vi "Record and playback example for pco.cameras with CamRam.vi"() -> ()   [LabVIEW 2012]
doc: "A short program to demonstrate the fundamentals of control and image acquision for pco.camera models with internal camRAM memory, such as the pco.dimax or pco.1200. The program records a sequence of images, with \"live\" updating, until the \"StopRecording\" button is pressed. A subset of recorded images is then read out from the camera RAM. WARNING: Limit the number of images read back tfrom the camera RAM to a reasonable number. Images are stored as a three-dimensional array, which can very large. Use ctrl-H for more help on the individual controls and indicators."
panel:
  in  "Rate":i32(ring) items=["12000000", "24000000"]
  out "bClose":bool
  in  "Quit":bool
  in  "ImageNr":i32
  in  "Image":i32
  out "BufNr1":i16
  out "BufNr0":i16
  in  "bUseBuffer1":bool
  in  "bUseBuffer0":bool
  in  "ROIX1":u16=1 min=1
  in  "ROIY1":u16=1 min=1
  in  "ROIY0":u16=1 min=1
  in  "ROIX0":u16=1 min=1
  out "Bits/pixel":u16
  in  "Readout":bool
  in  "Record":bool
  in  "Stop":u32=10 min=1
  in  "Start":u32=1 min=1
  in  "DelayTimeBase":u16(ring)=2 items=["nanoseconds", "microseconds", "milliseconds"]
  in  "ExposureTimeBase":u16(ring)=2 items=["nanoseconds", "microseconds", "milliseconds"]
  in  "Exposure":u32=10
  in  "Delay":u32
  out "Reading":bool
  in  "StorageMode":bool
  out "ImageCount":u32
  out "Image":u16[][](graph)
  in  "TriggerMode":u16(ring) items=["Auto", "Software", "External sequence start ", "External exposure control"]
  # "A short program to demonstrate the fundamentals of control and image acquision for pco.camera models with internal camRAM memory, such as the pco.dimax or pco.1200. The program records a sequence of images, with \"live\" updating, until the \"StopRecording\" button is pressed. A subset of recorded images is then read out from the camera RAM. WARNING: Limit the number of images read back tfrom the camera RAM to a reasonable number. Images are stored as a three-dimensional array, which can very large.  Use ctrl-H for more help on the individual controls and indicators."
  # "pco.labview"
  # "1) Setup camera:"
  # "FIFO"
  # "Recorder"
  # "2) Record  images:"
  # "3) Read out images:"
  # "4) Display image:"
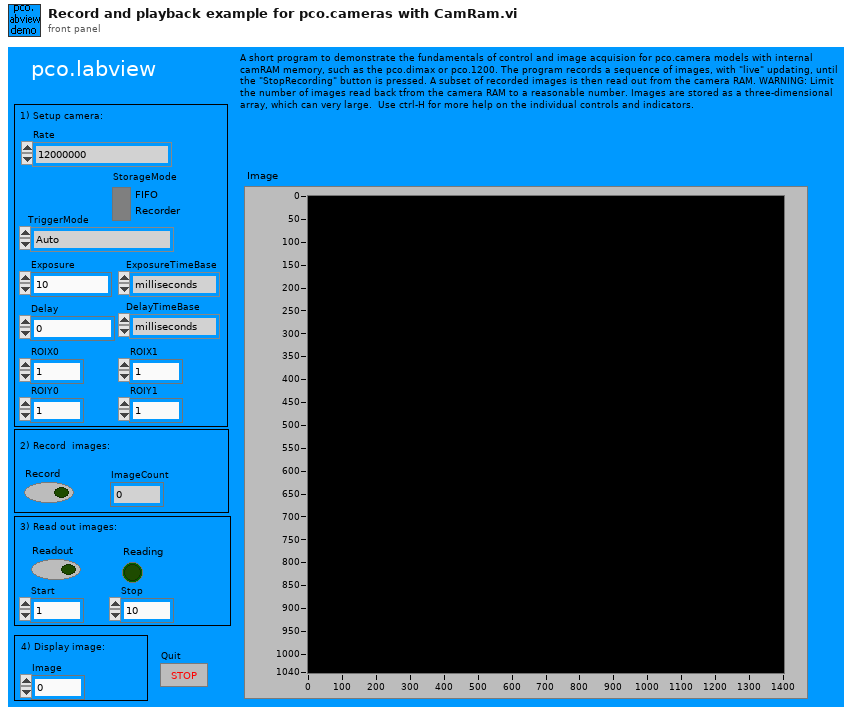
[diagram p1: front panel]
types:
  T1 = cluster{"SSize":u16, "CamType":u16, "CamsSubType":u16, "SerialNumber":u32, "HWVersion":u32, "FWVersion ":u32, "InterfaceType":u16, "HardwareVersions":cluster{"Board":u16, cluster{"string":string, "BatchNumber":u16, "MinorRevision":u8, "MajorRevision":u8, "Variant":u16}[]}, "FirmwareVersions":cluster{"DeviceNum":u16, cluster{"string":string, "MinorRevision":u8, "MajorRevision":u8, "Variant":u16}[]}}
  T2 = cluster{"Size":u16, "SensorTypeDESC":u16, "SensorSubtypeDESC":u16, "MaxHorizontalResStdDESC":u16, "MaxVerticalResStdDESC":u16, "MaxHorizontalResExtDESC":u16, "MaxVerticalResExtDESC":u16, "DynResDESC":u16, "MaxBinHorzDESC":u16, "BinHorzStepDESC":bool, "MaxBinVertDESC":u16, "BinVertStepDESC":bool, "ROIHorzStepDESC":u16, "ROIVertStepDESC":u16, "NumADCDESC":u16, "IRDESC":bool, "MinDelayDESC":u32, "MaxDelayDESC":u32, "MinDelayStepDESC":u32, "MinExpoDESC":u32, "MaxExpoDESC":u32, "MinExpoStepDESC":u32, "MinDelayIRDESC":u32, "MaxDelayIRDESC":u32, "MinExpoIRDESC":u32, "MaxExpoIRDESC":u32, "TimeTableDESC":bool, "DoubleImageDESC":bool, "MinCoolSetDESC":i16, "MaxCoolSetDESC":i16, "MDefaultCoolSetDESC":i16, "PowerDownModeDESC":bool, "OffsetRegDESC":bool, "ColorPattern":cluster{"UpperLeftColor":u8, "UpperRightColor":u8, "LowerLeftColor":u8, "LowerRightColor":u8}, "PatternTypeDESC":bool, "PixelRates":u32[], "CoversionFactors":u16[], "Reserved":u32[], "GeneralCapabilities":u32, "GeneralCapabilities 2":u32, "Min Size Hor":u16, "Min Size Vert":u16, "Ext Synch Freq":u32[], "Cooling Setpoints":i16[], "Soft ROI Hor Step":u16, "Soft ROI Vert Step":u16}
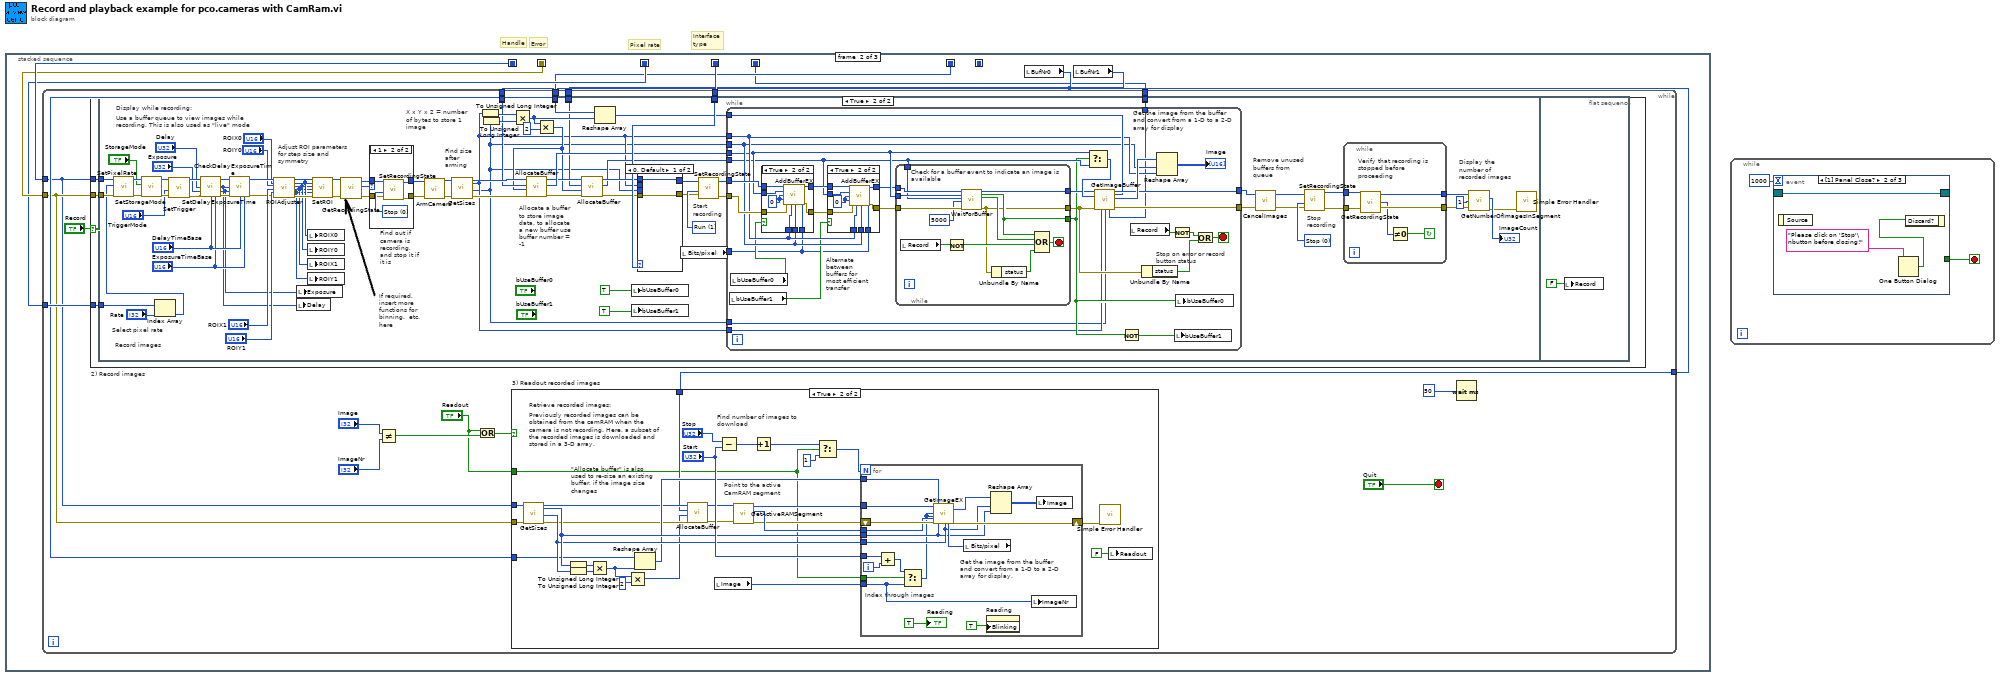
[diagram p0: block diagram]
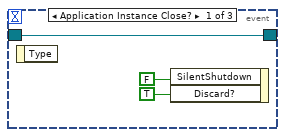
[diagram p2: hidden frame]
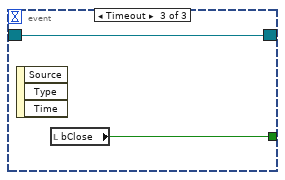
[diagram p3: hidden frame]
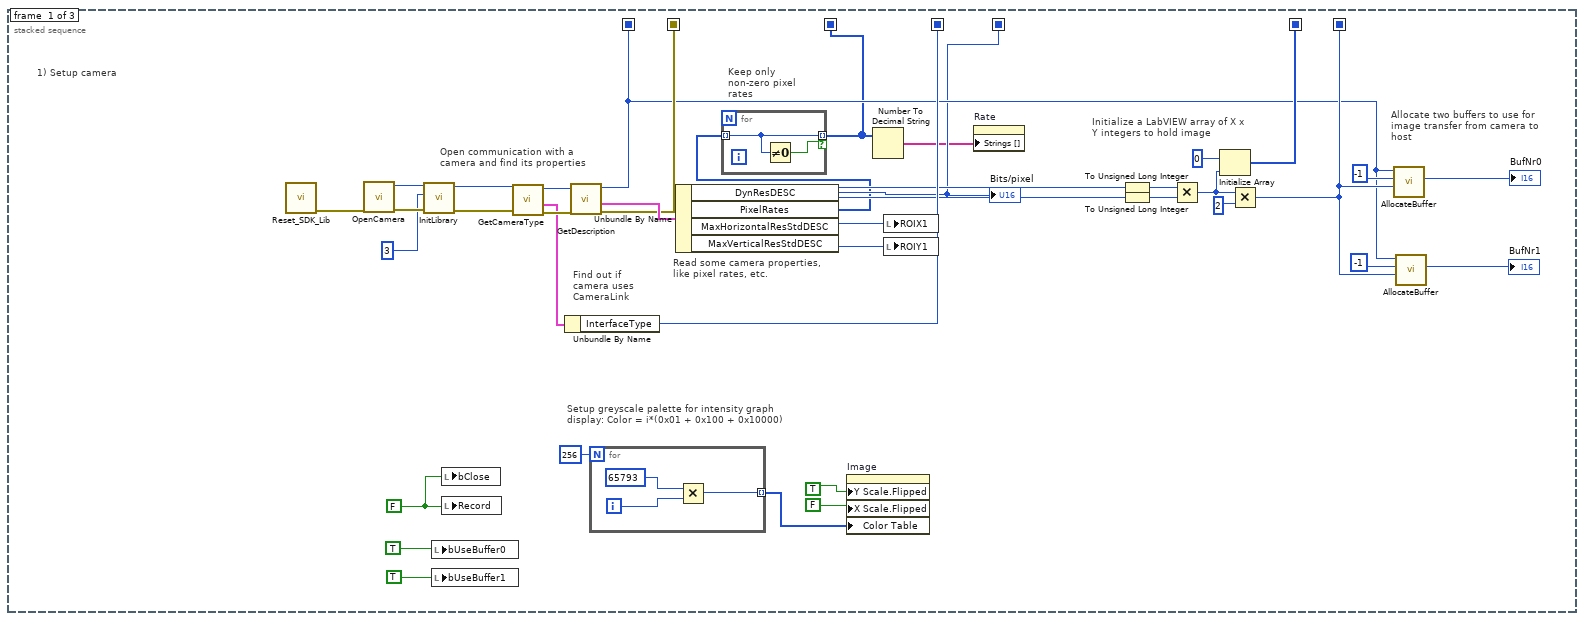
[diagram p4: hidden frame]
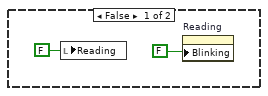
[diagram p5: hidden frame]
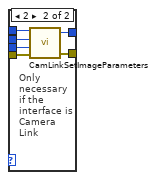
[diagram p9: hidden frame]
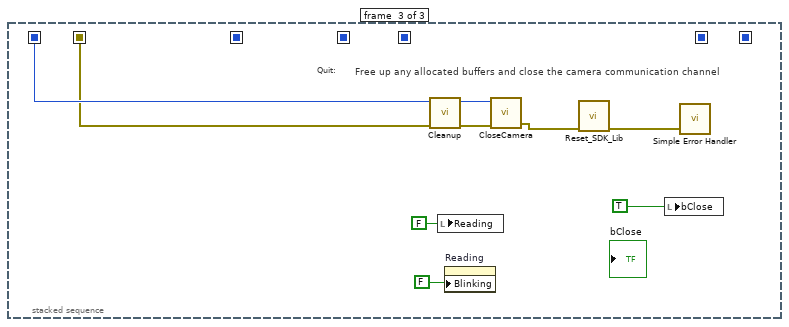
[diagram p11: hidden frame]
diagram:
  # "Interface type"
  # "Error"
  # "Handle"
  # "Pixel rate"
  n1 = stacked-sequence {
    seq-local: [w31 _ _] -> [_ w46 _]
    seq-local: [w18 _ _] -> [_ _ _]
    seq-local: [w1 _ _] -> [_ w48 _]
    seq-local: [w17 _ _] -> [_ w50 w299]
    seq-local: [w25 _ _] -> [_ w49 w298]
    seq-local: [w24 _ _] -> [_ w47 _]
    seq-local: [w4 _ _] -> [_ w43 _]
    frame #0 {
      w11 = FALSE ("stop")
      # "Keep only non-zero pixel rates"
      # "Read some camera properties, like pixel rates, etc."
      # "Allocate two buffers to use for image transfer from camera to host"
      # "1) Setup camera"
      # "Find out if camera uses CameraLink"
      # "Setup greyscale palette for intensity graph display: Color = i*(0x01 + 0x100 + 0x10000)"
      # "Initialize a LabVIEW array of X x Y integers to hold image"
      # "Open communication with a camera and find its properties"
      n2 = call "Reset_SDK_Lib.vi"() -> ("ErrorOut"=w7:errorcluster)  [unwired: 11 in]
      n3 = call "OpenCamera.vi"("ErrorIn"=w7) -> ("ErrorOut"=w9:errorcluster, "Handle out"=w10:u64)  [unwired: 3 in, 2 out]
      n4 = call "InitLibrary.vi"("error in (no error)"=w9, "InterfaceType"=u32 3, "ph"=w10) -> ("error out"=w5:errorcluster, "hout"=w6:u64)  [unwired: 7 in]
      n5 = local write "bUseBuffer0"(TRUE) -> ()
      n6 = local write "bUseBuffer1"(TRUE) -> ()
      n7 = local write "bClose"(w11) -> ()
      n8 = local write "Record"(w11) -> ()
      n9 = call "GetCameraType.vi"("ph"=w6, "error in (no error)"=w5) -> ("hout"=w28:u64, "CameraType"=w26:T1, "error out"=w27:errorcluster)  [unwired: 1 in, 1 out]
      n10 = Unbundle By Name(w26) -> ("InterfaceType"=w24:u16)
      n11 = call "GetDescription.vi"("ErrorIn"=w27, "ph"=w28) -> ("ErrorOut"=w25:errorcluster, "Description"=w30:T2, "hout"=w17:u64)  [unwired: 2 in, 1 out]
      n12 = for {
        N: 256 -> [_]
        tunnel: [w40] -> w34 mode=indexing
        i -> [w41]
        n13 = Multiply(x=65793, y=w41) -> (x*y=w40:i32)
      }
      n14 = Unbundle By Name(w30) -> ("DynResDESC"=w4:u16, "PixelRates"=w2:u32[], "MaxHorizontalResStdDESC"=w23:u16, "MaxVerticalResStdDESC"=w22:u16)
      "Bits/pixel" <- w4
      n15 = for {
        tunnel: w2 -> [w39] mode=indexing
        tunnel: [w39] -> w1 mode=indexing if=w38
        n16 = Not Equal To 0?(x=w39) -> (x != 0?=w38:bool)
      }
      n17 = property on="Image" class="IntGraph (strict)"("Y Scale.Flipped"=TRUE, "X Scale.Flipped"=FALSE, "Color Table"=w34) -> ()  [unwired: 2 in, 2 out]
      n18 = Number To Decimal String(number=w1) -> (decimal integer string=w3:string[])  [unwired: 1 in]
      n19 = local write "ROIX1"(w23) -> ()
      n20 = local write "ROIY1"(w22) -> ()
      n21 = property on="Rate" class="Ring (strict)"("Strings []"=w3) -> ()  [unwired: 2 in, 2 out]
      n22 = To Unsigned Long Integer(number=w23) -> (unsigned 32bit integer=w20:u32)
      n23 = To Unsigned Long Integer(number=w22) -> (unsigned 32bit integer=w19:u32)
      n24 = Multiply(x=w20, y=w19) -> (x*y=w32:u32)
      n25 = Initialize Array(u16 0 ("Element Data"), w32) -> (w31:u16[])
      n26 = Multiply(x=w32, y=u32 2) -> (x*y=w18:u32)
      n27 = call "AllocateBuffer.vi"("Size"=w18, "BufNr"=i16 -1, "ph"=w17) -> ("BufNrOut"=→"BufNr0":i16)  [unwired: 3 in, 5 out]
      n28 = call "AllocateBuffer.vi"("Size"=w18, "BufNr"=-1, "ph"=w17) -> ("BufNrOut"=→"BufNr1":i16)  [unwired: 3 in, 5 out]
    }
    frame #1 {
      n29 = local read "BufNr0"() -> (w45:i16)
      n30 = local read "BufNr1"() -> (w44:i16)
      n31 = while {
        tunnel: w45 -> [w60]
        tunnel: w45 -> [w61]
        tunnel: w46 -> [w63]
        tunnel: w47 -> [w64]
        tunnel: w48 -> [w65]
        tunnel: w49 -> [w62]
        tunnel: w50 -> [w58]
        tunnel: w44 -> [w59]
        tunnel: w43 -> [w51]
        stop <- "Quit" stop-if-true
        n32 = case "2) Record images" shown="True" "Record" {
          tunnel: w58 -> [_ w124]
          tunnel: w62 -> [_ w123]
          tunnel: w65 -> [_ w122]
          tunnel: w64 -> [_ w121]
          tunnel: w63 -> [_ w120]
          tunnel: w61 -> [_ w119]
          tunnel: w59 -> [_ w118]
          tunnel: w51 -> [_ w117]
          frame False {
          }
          frame True {
            n33 = flat-sequence {
              tunnel: w124 -> [w186]
              tunnel: w123 -> [w185]
              tunnel: w122 -> [w147]
              tunnel: w121 -> [w183]
              tunnel: w120 -> [w181]
              tunnel: w119 -> [w171]
              tunnel: w118 -> [w165]
              tunnel: w117 -> [w149]
              frame #0 {
                w204 = u16 1 items=["Stop", "Run"] ("RecordingState")
                w207 = u16 0 items=["Stop", "Run"] ("RecordingState")
                # "Adjust ROI parameters   for step size and symmetry"
                # "Select pixel rate"
                # "Remove unused buffers from queue"
                # "Display the number of recorded images"
                # "Record images"
                # "Start recording"
                # "Allocate a buffer to store image data. to allocate a new buffer use buffer number = -1"
                # "Find size after arming"
                # "Find out if camera is recording, and stop it if it is"
                # "If required, insert more functions for binning.  etc. here"
                # "X x Y x 2 = number of bytes to store 1 image"
                # "Stop recording"
                # "Use a buffer queue to view images while recording. This is also used as \"live\" mode"
                # "Display while recording:"
                n34 = Index Array(array=w147, index="Rate") -> (element=w146:u32)
                n35 = call "SetPixelRate.vi"("error in (no error)"=w185, "PixelRate"=w146, "ph"=w186) -> ("error out"=w202:errorcluster, "hout"=w203:u64)  [unwired: 2 in, 1 out]
                n36 = call "SetStorageMode.vi"("error in (no error)"=w202, "StorageMode"="StorageMode", "ph"=w203) -> ("error out"=w194:errorcluster, "hout"=w195:u64)  [unwired: 2 in, 1 out]
                n37 = call "SetTrigger.vi"("error in (no error)"=w194, "TriggerMode"="TriggerMode", "ph"=w195) -> ("error out"=w134:errorcluster, "hout"=w131:u64)  [unwired: 2 in, 1 out]
                n38 = call "CheckDelayExposureTime.vi"("ph"=w131, "Delay"="Delay", "Exposure"="Exposure", "error in (no error)"=w134, "DelayTimeBase"="DelayTimeBase", "ExposureTimeBase"="ExposureTimeBase") -> ("hout"=w132:u64, "Delay Out"=w126:u32, "Exposure Out"=w125:u32, "error out"=w133:errorcluster)  [unwired: 4 in, 2 out]
                n39 = call "SetDelayExposureTime.vi"("ph"=w132, "Delay"=w126, "Exposure"=w125, "error in (no error)"=w133, "DelayTimeBase"="DelayTimeBase", "ExposureTimeBase"="ExposureTimeBase") -> ("hout"=w174:u64, "error out"=w140:errorcluster)  [unwired: 7 in, 1 out]
                n40 = call "ROIAdjuster.vi"("HandleIn"=w174, "ROIXmin"="ROIX0", "ROIYmin"="ROIY0", "ROIXmax"="ROIX1", "ROIYmax"="ROIY1", "ErrorIn"=w140) -> ("hout"=w145:u64, "ROIX0Mod"=w138:u16, "ROIY0Mod"=w137:u16, "ROIX1Mod"=w136:u16, "ROIY1Mod"=w135:u16, "ErrorOut"=w139:errorcluster)  [unwired: 7 in, 1 out]
                n41 = local write "Delay"(w126) -> ()
                n42 = local write "Exposure"(w125) -> ()
                n43 = local write "ROIX0"(w138) -> ()
                n44 = local write "ROIY0"(w137) -> ()
                n45 = local write "ROIX1"(w136) -> ()
                n46 = local write "ROIY1"(w135) -> ()
                n47 = call "SetROI.vi"("ph"=w145, "ROIX0"=w138, "ROIY0"=w137, "ROIX1"=w136, "ROIY1"=w135, "error in (no error)"=w139) -> ("hout"=w173:u64, "error out"=w172:errorcluster)  [unwired: 12 in]
                n48 = call "GetRecordingState.vi"("ErrorIn"=w172, "ph"=w173) -> ("ErrorOut"=w198:errorcluster, "RecordingState"=w200:u16, "hout"=w199:u64)  [unwired: 2 in, 1 out]
                n49 = case shown="1" w200 {
                  tunnel: w199 -> [w288 w292]
                  tunnel: w198 -> [w287 w291]
                  tunnel: [w288 w290] -> w197
                  tunnel: [w287 w289] -> w196
                  frame 0, Default {
                  }
                  frame 1 {
                    w293 = u16 0 items=["Stop", "Run"] ("RecordingState")
                    n50 = call "SetRecordingState.vi"("ErrorIn"=w291, "RecordingState"=w293, "ph"=w292) -> ("ErrorOut"=w289:errorcluster, "hout"=w290:u64)  [unwired: 2 in, 1 out]
                  }
                }
                n51 = call "ArmCamera.vi"("error in (no error)"=w196, "ph"=w197) -> ("error out"=w192:errorcluster, "hout"=w193:u64)  [unwired: 1 in, 1 out]
                n52 = call "GetSizes.vi"("ph"=w193, "ErrorIn"=w192) -> ("hout"=w189:u64, "XResAct"=w151:u16, "YResAct"=w150:u16, "ErrorOut"=w191:errorcluster)  [unwired: 11 in, 3 out]
                n53 = To Unsigned Long Integer(number=w151) -> (unsigned 32bit integer=w175:u32)
                n54 = To Unsigned Long Integer(number=w150) -> (unsigned 32bit integer=w176:u32)
                n55 = Multiply(x=w175, y=w176) -> (x*y=w177:u32)
                n56 = Multiply(x=w177, y=u32 2) -> (x*y=w166:u32)
                n57 = call "AllocateBuffer.vi"("error in (no error)"=w191, "Size"=w166, "BufNr"=w171, "ph"=w189) -> ("error out"=w170:errorcluster, "BufNrOut"=w178:i16, "hout"=w168:u64)  [unwired: 2 in, 3 out]
                n58 = call "AllocateBuffer.vi"("error in (no error)"=w170, "Size"=w166, "BufNr"=w165, "ph"=w168) -> ("error out"=w169:errorcluster, "BufNrOut"=w164:i16, "hout"=w167:u64)  [unwired: 2 in, 3 out]
                n59 = Reshape Array(w181, w177) -> (w180:u16[])
                n60 = local write "bUseBuffer0"(TRUE) -> ()
                n61 = local write "bUseBuffer1"(TRUE) -> ()
                n62 = case shown="0, Default" w183 {
                  tunnel: w169 -> [w279 w286]
                  tunnel: [w279 w285] -> w188
                  tunnel: w167 -> [w280 w284]
                  tunnel: [w280 w283] -> w187
                  tunnel: w150 -> [_ w282]
                  tunnel: w151 -> [_ w281]
                  frame 0, Default {
                  }
                  frame 2 {
                    # "Only necessary if the interface is Camera Link"
                    n63 = call "CamLinkSetImageParameters.vi"("error in (no error)"=w286, "YRes"=w282, "XRes"=w281, "ph"=w284) -> ("error out"=w285:errorcluster, "hout"=w283:u64)  [unwired: 1 out]
                  }
                }
                n64 = local read "Bits/pixel"() -> (w157:u16)
                n65 = call "SetRecordingState.vi"("ErrorIn"=w188, "RecordingState"=w204, "ph"=w187) -> ("ErrorOut"=w184:errorcluster, "hout"=w182:u64)  [unwired: 2 in, 1 out]
                n66 = while {
                  tunnel: w178 -> [w220]
                  tunnel: w180 -> [w233]
                  tunnel: w182 -> [w232]
                  tunnel: w150 -> [w227]
                  tunnel: w151 -> [w228]
                  tunnel: w184 -> [w230]
                  tunnel: [w235] -> w156
                  tunnel: [w236] -> w155
                  tunnel: w164 -> [w219]
                  tunnel: w157 -> [w223]
                  tunnel: w151 -> [w210]
                  tunnel: w150 -> [w209]
                  tunnel: w149 -> [w208]
                  stop <- w211 stop-if-true
                  # "Alternate between buffers for most efficient transfer"
                  # "Stop on error or record button status"
                  # "Get the image from the buffer and convert from a 1-D to a 2-D array for display"
                  n67 = local read "bUseBuffer1"() -> (w225:bool)
                  n68 = local read "bUseBuffer0"() -> (w226:bool)
                  n69 = case shown="True" w226 {
                    tunnel: [w239 w248] -> w229
                    tunnel: [w238 w247] -> w231
                    tunnel: w220 -> [_ w246]
                    tunnel: w232 -> [w238 w245]
                    tunnel: w223 -> [_ w243]
                    tunnel: w228 -> [_ w242]
                    tunnel: w227 -> [_ w241]
                    tunnel: w230 -> [w239 w240]
                    frame False {
                    }
                    frame True {
                      w244 = 0
                      n70 = call "AddBufferEX.vi"("ph"=w245, "BuffNr"=w246, "1stImage"=w244, "LastImage"=w244, "error in (no error)"=w240, "XRes"=w242, "YRes"=w241, "BitPerPixel"=w243) -> ("hout"=w247:u64, "error out"=w248:errorcluster)  [unwired: 5 in, 1 out]
                    }
                  }
                  n71 = case shown="True" w225 {
                    tunnel: [w249 w259] -> w217
                    tunnel: [w250 w258] -> w218
                    tunnel: w219 -> [_ w257]
                    tunnel: w231 -> [w250 w256]
                    tunnel: w223 -> [_ w254]
                    tunnel: w228 -> [_ w253]
                    tunnel: w227 -> [_ w252]
                    tunnel: w229 -> [w249 w251]
                    frame False {
                    }
                    frame True {
                      w255 = 0
                      n72 = call "AddBufferEX.vi"("ph"=w256, "BuffNr"=w257, "1stImage"=w255, "LastImage"=w255, "error in (no error)"=w251, "XRes"=w253, "YRes"=w252, "BitPerPixel"=w254) -> ("hout"=w258:u64, "error out"=w259:errorcluster)  [unwired: 5 in, 1 out]
                    }
                  }
                  n73 = while {
                    tunnel: w220 -> [w267]
                    tunnel: w219 -> [w266]
                    tunnel: w218 -> [w269]
                    tunnel: w217 -> [w268]
                    tunnel: [w265] -> w216
                    tunnel: [w261] -> w214
                    tunnel: [w264] -> w215
                    stop <- w270 stop-if-true
                    # "Check for a buffer event to indicate an image is available"
                    n74 = local read "Record"() -> (w272:bool)
                    n75 = Not(x=w272) -> (.not. x?=w271:bool)
                    n76 = call "WaitForBuffer.vi"("ph"=w269, "sBufNr"=w267, "sBufNr 2"=w266, "timeout"=5000, "error in (no error)"=w268) -> ("hout"=w265:u64, "Buffer_Ready"=w264:bool, "Buffer_Ready 2"=w263:bool, "error out"=w261:errorcluster)  [unwired: 10 in, 1 out]
                    n77 = Unbundle By Name(w261) -> ("status"=w260:bool)
                    n78 = Compound Arithmetic op=OR(w264, w263, w271, w260) -> (w270:bool)
                  }
                  n79 = Select(t=w220, s=w215, f=w219) -> (s? t:f=w224:i16)
                  n80 = call "GetImageBuffer.vi"("ph"=w216, "BuffIn"=w233, "BuffNr"=w224, "error in (no error)"=w214, "xRes"=w210, "yRes"=w209, "Bitresolution"=w208) -> ("hout"=w235:u64, "BuffOut"=w237:u16[], "error out"=w236:errorcluster)  [unwired: 5 in, 1 out]
                  n81 = Not(x=w215) -> (.not. x?=w222:bool)
                  n82 = local read "Record"() -> (w234:bool)
                  n83 = Unbundle By Name(w214) -> ("status"=w212:bool)
                  n84 = Reshape Array(w237, w227, w228) -> (→"Image":u16[][])
                  n85 = Not(x=w234) -> (.not. x?=w213:bool)
                  n86 = local write "bUseBuffer1"(w222) -> ()
                  n87 = local write "bUseBuffer0"(w215) -> ()
                  n88 = Or(x=w213, y=w212) -> (x .or. y?=w211:bool)
                }
                n89 = call "CancelImages.vi"("error in (no error)"=w155, "ph"=w156) -> ("error out"=w161:errorcluster, "hout"=w160:u64)  [unwired: 1 in, 1 out]
                n90 = call "SetRecordingState.vi"("ErrorIn"=w161, "RecordingState"=w207, "ph"=w160) -> ("ErrorOut"=w205:errorcluster, "hout"=w206:u64)  [unwired: 2 in, 1 out]
                n91 = while {
                  tunnel: [w276] -> w154
                  tunnel: w205 -> [w277]
                  tunnel: w206 -> [w278]
                  tunnel: [w273] -> w153
                  stop <- w274 continue-if-true
                  # "Verify that recording is stopped before proceeding"
                  n92 = call "GetRecordingState.vi"("ErrorIn"=w277, "ph"=w278) -> ("ErrorOut"=w276:errorcluster, "RecordingState"=w275:u16, "hout"=w273:u64)  [unwired: 2 in, 1 out]
                  n93 = Not Equal To 0?(x=w275) -> (x != 0?=w274:bool)
                }
                n94 = call "GetNumberOfImagesInSegment.vi"("ph"=w153, "Segment"=u16 1, "error in (no error)"=w154) -> ("ValidImageCnt"=→"ImageCount":u32, "error out"=w152:errorcluster)  [unwired: 3 out]
                n95 = call <vilib>:"Simple Error Handler.vi"("error in (no error)"=w152) -> ()  [unwired: 4 in, 5 out]
              }
              frame #1 {
                n96 = local write "Record"(FALSE ("Record")) -> ()
              }
            }
          }
        }
        n97 = Not Equal?(x="Image", y="ImageNr") -> (x != y?=w55:bool)
        n98 = Or(x="Readout", y=w55) -> (x .or. y?=w54:bool)
        n99 = case "3) Readout recorded images" shown="True" w54 {
          tunnel: w63 -> [_ w91]
          tunnel: w58 -> [_ w83]
          tunnel: w62 -> [_ w82]
          tunnel: w60 -> [_ w76]
          tunnel: "Readout" -> [_ w70]
          frame False {
            n100 = local write "Reading"(FALSE ("Reading")) -> ()
            n101 = property on="Reading" class="Bool (strict)"("Blinking"=FALSE) -> ()  [unwired: 2 in, 2 out]
          }
          frame True {
            # "Point to the active CamRAM segment"
            # "\"Allocate buffer\" is also used to re-size an existing buffer, if the image size changes"
            # "Find number of images to download"
            # "Previously recorded images can be obtained from the camRAM when the camera is not recording. Here, a subset of the recorded images is downloaded and stored in a 3-D array."
            # "Retrieve recorded images:"
            n102 = call "GetSizes.vi"("ph"=w83, "ErrorIn"=w82) -> ("hout"=w89:u64, "XResAct"=w93:u16, "YResAct"=w92:u16, "ErrorOut"=w87:errorcluster)  [unwired: 11 in, 3 out]
            n103 = To Unsigned Long Integer(number=w93) -> (unsigned 32bit integer=w79:u32)
            n104 = To Unsigned Long Integer(number=w92) -> (unsigned 32bit integer=w80:u32)
            n105 = Multiply(x=w79, y=w80) -> (x*y=w81:u32)
            n106 = Multiply(x=w81, y=u32 2) -> (x*y=w78:u32)
            n107 = Reshape Array(w91, w81) -> (w90:u16[])
            n108 = call "AllocateBuffer.vi"("error in (no error)"=w87, "Size"=w78, "BufNr"=w76, "ph"=w89) -> ("error out"=w86:errorcluster, "hout"=w88:u64)  [unwired: 2 in, 4 out]
            n109 = local read "Image"() -> (w74:i32)
            n110 = Subtract(x="Stop", y="Start") -> (x-y=w97:u32)
            n111 = call "GetActiveRAMSegment.vi"("error in (no error)"=w86, "ph"=w88) -> ("error out"=w84:errorcluster, "ActSeg"=w94:u16, "hout"=w85:u64)  [unwired: 2 in, 1 out]
            n112 = Increment(x=w97) -> (x+1=w73:u32)
            n113 = Select(t=w73, s=w70, f=1) -> (s? t:f=w72:u32)
            n114 = for {
              N: w72 -> [_]
              tunnel: w85 -> [w116]
              shift-right: [w113] -> w75
              shift-left: w84 -> [w112]
              tunnel: "Start" -> [w109]
              tunnel: w94 -> [w107]
              tunnel: w93 -> [w103]
              tunnel: w92 -> [w104]
              tunnel: w90 -> [w105]
              tunnel: w74 -> [w99]
              tunnel: w70 -> [w101]
              i -> [w108]
              # "Get the image from the buffer and convert from a 1-D to a 2-D array for display."
              # "Index through images"
              n115 = Add(x=w109, y=w108) -> (x+y=w100:u32)
              n116 = Select(t=w100, s=w101, f=w99) -> (s? t:f=w102:u32)
              n117 = local read "Bits/pixel"() -> (w106:u16)
              n118 = call "GetImageEX.vi"("ph"=w116, "1stImage"=w102, "lastImage"=w102, "segment"=w107, "error in (no error)"=w112, "BuffIn"=w105, "xRes"=w103, "yRes"=w104, "BitPerPixel"=w106) -> ("BuffOut"=w115:u16[], "error out"=w113:errorcluster)  [unwired: 7 in, 2 out]
              n119 = property on="Reading" class="Bool (strict)"("Blinking"=TRUE) -> ()  [unwired: 2 in, 2 out]
              n120 = Reshape Array(w115, w104, w103) -> (w114:u16[][])
              n121 = local write "ImageNr"(w99) -> ()
              n122 = local write "Image"(w114) -> ()
              "Reading" <- TRUE ("Reading")
            }
            n123 = call <vilib>:"Simple Error Handler.vi"("error in (no error)"=w75) -> ()  [unwired: 4 in, 5 out]
            n124 = local write "Readout"(FALSE ("Readout")) -> ()
          }
        }
        n125 = Wait (ms)(milliseconds to wait=u32 50) -> ()  [unwired: 1 out]
      }
    }
    frame #2 {
      # "Free up any allocated buffers and close the camera communication channel"
      # "Quit:"
      n126 = call "Cleanup.vi"("error in (no error)"=w298, "ph"=w299) -> ("error out"=w297:errorcluster, "hout"=w296:u64)  [unwired: 8 in]
      n127 = local write "Reading"(FALSE ("Reading")) -> ()
      n128 = property on="Reading" class="Bool (strict)"("Blinking"=FALSE) -> ()  [unwired: 2 in, 2 out]
      n129 = call "CloseCamera.vi"("ErrorIn"=w297, "Handle in"=w296) -> ("ErrorOut"=w295:errorcluster)  [unwired: 1 in, 2 out]
      n130 = call "Reset_SDK_Lib.vi"("ErrorIn"=w295) -> ("ErrorOut"=w300:errorcluster)  [unwired: 10 in]
      n131 = local write "bClose"(TRUE) -> ()
      n132 = call <vilib>:"Simple Error Handler.vi"("error in (no error)"=w300) -> ()  [unwired: 4 in, 5 out]
    }
  }
  n133 = while {
    stop <- w304 stop-if-true
    n134 = event shown="[1] Panel Close?" {
      selector: _ -> [w306 w311 w313]
      dyn-events: [w306 w311 w313] -> _
      timeout: 1000 -> [_ _ _]
      tunnel: [_ _ w312] -> w304
      event Application Instance Close? {
        n135 = event-data() -> ()  [unwired: 1 in, 1 out]
        n136 = event-data("SilentShutdown"=FALSE, "Discard?"=TRUE) -> ()  [unwired: 1 in, 1 out]
      }
      event Panel Close? {
        n137 = event-data() -> ()  [unwired: 1 in, 1 out]
        n138 = One Button Dialog(message="Please click on 'Stop'\nbutton before closing!") -> (true=w309:bool)  [unwired: 1 in]
        n139 = event-data("Discard?"=w309) -> ()  [unwired: 1 in, 1 out]
      }
      event Timeout {
        n140 = event-data() -> ()  [unwired: 1 in, 3 out]
        n141 = local read "bClose"() -> (w312:bool)
      }
    }
  }
